vi "Build One Term Numeric Functions.vi"(8 "Names":string[](array[string]), 9 "Representation":T1[](array[typedef]), 10 "Abstract Type Locations":string[](array[string]), 11 "Comparison Name":string) -> ()   [LabVIEW 2019]
uses:
  4dc09652-b8df-42b5-b160-fe6468400f37.vi
  <vilib>/numeric/LVNumericRepresentation.ctl
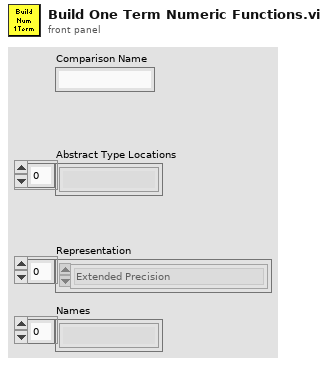
[diagram p1: front panel]
types:
  T1 = typedef "LVNumericRepresentation.ctl" = enum32{"Extended Precision", "Double Precision", "Single Precision", "Long", "Word", "Byte", "Unsigned Long", "Unsigned Word", "Unsigned Byte", "Complex Extended", "Complex Double", "Complex Single", "Quad", "Unsigned Quad", "Fixed-Point"}
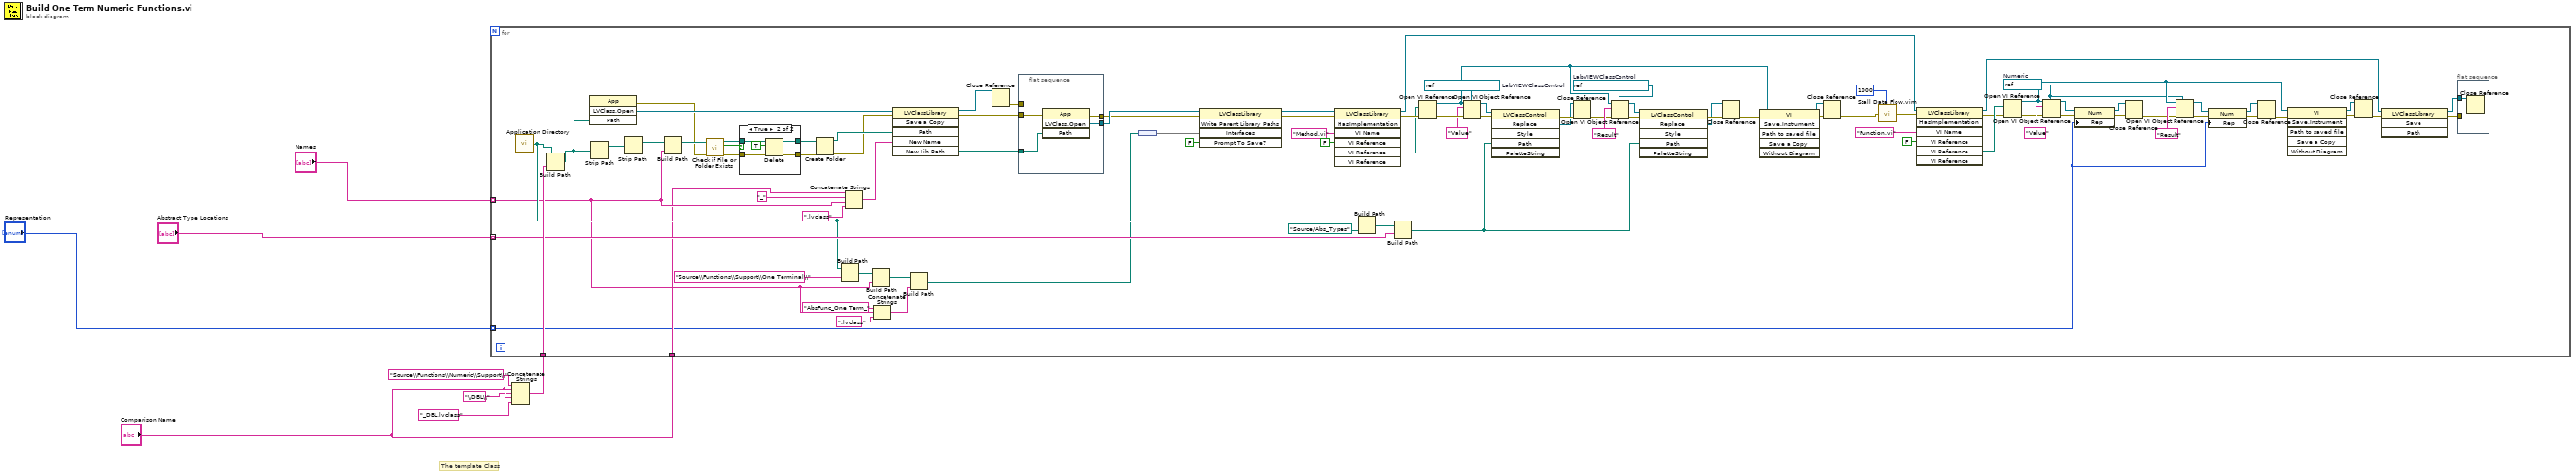
[diagram p0: block diagram]
diagram:
  # "The template Class"
  n1 = Concatenate Strings("Source\\Functions\\Numeric\\Support\\", "Comparison Name", "\\DBL\\", "Comparison Name", "_DBL.lvclass") -> (w7:string)
  n2 = for {
    tunnel: "Names" -> [w43] mode=indexing
    tunnel: w7 -> [w82]
    tunnel: "Abstract Type Locations" -> [w74] mode=indexing
    tunnel: "Representation" -> [w11] mode=indexing
    tunnel: "Comparison Name" -> [w31]
    w22 = refnum<vi> refnum  # LabVIEWClassControl
    w10 = refnum<vi> refnum  # Numeric
    w69 = refnum<vi> refnum  # LabVIEWClassControl
    n3 = call <vilib>:"Application Directory.vi"() -> ("Application Directory"=w47:path)
    n4 = Build Path(base path=w47, name or relative path=w82) -> (appended path=w83:path)
    n5 = invoke class="App" method="LVClass.Open"("Path"=w83) -> (error out=w88:errorcluster, "LVClass.Open"=w101:refnum<vi>)  [unwired: 3 in, 2 out]
    n6 = Strip Path(path=w83) -> (stripped path=w99:path)  [unwired: 1 out]
    n7 = Strip Path(path=w99) -> (stripped path=w98:path)  [unwired: 1 out]
    n8 = Build Path(base path=w98, name or relative path=w43) -> (appended path=w94:path)
    n9 = call <vilib>:"Check if File or Folder Exists.vi"("error in (no error)"=w88, "path"=w94) -> ("error out"=w87:errorcluster, "file or folder exists?"=w96:bool, "dup path"=w97:path)  [unwired: 7 in]
    n10 = case shown="True" w96 {
      tunnel: w97 -> [w108 w113]
      tunnel: [w108 w111] -> w95
      tunnel: w87 -> [w107 w110]
      tunnel: [w107 w109] -> w86
      frame False {
      }
      frame True {
        n11 = Delete(path (use dialog)=w113, entire hierarchy (F)=TRUE, error in=w110) -> (deleted path=w111:path, error out=w109:errorcluster)  [unwired: 2 in, 1 out]
      }
    }
    n12 = Create Folder(path (use dialog)=w95, error in=w86) -> (created path=w93:path, error out=w85:errorcluster)  [unwired: 1 in, 1 out]
    n13 = Build Path(base path=w47, name or relative path="Source\\Functions\\Support\\One Terminal\\") -> (appended path=w46:path)
    n14 = Concatenate Strings(w31, "_", w43, ".lvclass") -> (w81:string)
    n15 = Build Path(base path=w46, name or relative path=w43) -> (appended path=w45:path)
    n16 = Concatenate Strings("AbsFunc_One Term_" ("string"), w43, ".lvclass") -> (w41:string)
    n17 = invoke class="LVClassLibrary" method="Save a Copy"(reference=w101, error in=w85, "Path"=w93, "New Name"=w81) -> (reference out=w100:refnum<vi>, error out=w89:errorcluster, "New Lib Path"=w90:path)  [unwired: 2 in, 3 out]
    n18 = Build Path(base path=w45, name or relative path=w41) -> (appended path=w39:path)
    n19 = Close Reference(reference=w100) -> (error out=w84:errorcluster)  [unwired: 1 in]
    n20 = flat-sequence {
      tunnel: w90 -> [w105]
      tunnel: w89 -> [w106]
      tunnel: w84 -> [_]
      tunnel: [w103] -> w56
      tunnel: [w104] -> w40
      frame #0 {
        n21 = invoke class="App" method="LVClass.Open"(error in=w106, "Path"=w105) -> (error out=w104:errorcluster, "LVClass.Open"=w103:refnum<vi>)  [unwired: 2 in, 2 out]
      }
    }
    n22 = node(w39) -> (w38:set{path})
    n23 = invoke class="LVClassLibrary" method="Write Parent Library Paths"(reference=w56, error in=w40, "Interfaces"=w38, "Prompt To Save?"=FALSE) -> (reference out=w55:refnum<vi>, error out=w54:errorcluster)  [unwired: 1 in, 3 out]
    n24 = invoke class="LVClassLibrary" method="HasImplementation"(reference=w55, error in=w54, "VI Name"="Method.vi", "VI Reference"=FALSE ("Consider Parents?")) -> (reference out=w57:refnum<vi>, error out=w79:errorcluster, "VI Reference"=w78:path)  [unwired: 3 in, 4 out]
    n25 = Build Path(base path=w47, name or relative path=path "Source/Abs_Types") -> (appended path=w75:path)
    n26 = Build Path(base path=w75, name or relative path=w74) -> (appended path=w21:path)
    n27 = Open VI Reference(vi path=w78, error in (no error)=w79) -> (vi reference=w9:refnum<vi>, error out=w73:errorcluster)  [unwired: 4 in]
    n28 = Open VI Object Reference(7:w69, 8:w73, 10:"Value" ("name/order"), 11:w9) -> (0:w71:errorcluster, 3:w70:refnum<vi>)
    n29 = invoke class="LVClassControl" method="Replace"(reference=w70, error in=w71, "Path"=w21) -> (error out=w27:errorcluster, "Replace"=w26:refnum<vi>)  [unwired: 3 in, 4 out]
    n30 = Close Reference(reference=w26, error in (no error)=w27) -> (error out=w23:errorcluster)
    n31 = Open VI Object Reference(7:w22, 8:w23, 10:"Result" ("name/order"), 11:w9) -> (0:w29:errorcluster, 3:w30:refnum<vi>)
    n32 = invoke class="LVClassControl" method="Replace"(reference=w30, error in=w29, "Path"=w21) -> (error out=w25:errorcluster, "Replace"=w24:refnum<vi>)  [unwired: 3 in, 4 out]
    n33 = Close Reference(reference=w24, error in (no error)=w25) -> (error out=w20:errorcluster)
    n34 = invoke class="VI" method="Save.Instrument"(reference=w9, error in=w20) -> (reference out=w34:refnum<vi>, error out=w35:errorcluster)  [unwired: 4 in, 4 out]
    n35 = Close Reference(reference=w34, error in (no error)=w35) -> (error out=w60:errorcluster)
    n36 = call "Stall Data Flow.vim"("value in"=w60, "milliseconds to wait"=u32 1000) -> ("value out"=w59:errorcluster)  [unwired: 1 out]
    n37 = invoke class="LVClassLibrary" method="HasImplementation"(reference=w57, error in=w59, "VI Name"="Function.vi", "VI Reference"=FALSE ("Consider Parents?")) -> (reference out=w50:refnum<vi>, error out=w65:errorcluster, "VI Reference"=w66:path)  [unwired: 3 in, 4 out]
    n38 = Open VI Reference(vi path=w66, error in (no error)=w65) -> (vi reference=w15:refnum<vi>, error out=w63:errorcluster)  [unwired: 4 in]
    n39 = Open VI Object Reference(7:w10, 8:w63, 10:"Value" ("name/order"), 11:w15) -> (0:w36:errorcluster, 3:w37:refnum<vi>)
    n40 = property class="Num"(reference=w37, error in=w36, "Rep"=w11) -> (reference out=w61:refnum<vi>, error out=w62:errorcluster)
    n41 = Close Reference(reference=w61, error in (no error)=w62) -> (error out=w16:errorcluster)
    n42 = Open VI Object Reference(7:w10, 8:w16, 10:"Result" ("name/order"), 11:w15) -> (0:w19:errorcluster, 3:w12:refnum<vi>)
    n43 = property class="Num"(reference=w12, error in=w19, "Rep"=w11) -> (reference out=w13:refnum<vi>, error out=w18:errorcluster)
    n44 = Close Reference(reference=w13, error in (no error)=w18) -> (error out=w14:errorcluster)
    n45 = invoke class="VI" method="Save.Instrument"(reference=w15, error in=w14) -> (reference out=w33:refnum<vi>, error out=w32:errorcluster)  [unwired: 4 in, 4 out]
    n46 = Close Reference(reference=w33, error in (no error)=w32) -> (error out=w52:errorcluster)
    n47 = invoke class="LVClassLibrary" method="Save"(reference=w50, error in=w52) -> (reference out=w49:refnum<vi>, error out=w51:errorcluster)  [unwired: 2 in, 2 out]
    n48 = flat-sequence {
      tunnel: w49 -> [w102]
      tunnel: w51 -> [_]
      frame #0 {
        n49 = Close Reference(reference=w102) -> ()  [unwired: 1 in, 1 out]
      }
    }
  }
